vi "Configure System Time Stamp.vi"(7 "System Date Time":timestamp, 8 "error in (no error)":errorcluster, 9 "Time Stamp Format (0: Absolute)":i32(ring) items=["Absolute", "Delta"], 10 "Time Stamp Type (0: Relative-time)":i32(ring) items=["Relative-time", "Real-time"], 11 "VISA resource name":refnum<visa-resource-name>) -> (0 "error out":errorcluster, 3 "VISA resource name out":refnum<visa-resource-name>)   [LabVIEW 2020, in "Keithley 6517.lvlib"]
doc: "Configures time stamps.\n\nNote:\nFor relative-time time stamp, uses the values to set it only when disable reset relative time stamp.\n\nThis VI is <B>NOT</B> compatible with model <B>6514</B>."
uses:
  <instrlib>/Keithley 6517/Keithley 6517.lvlib
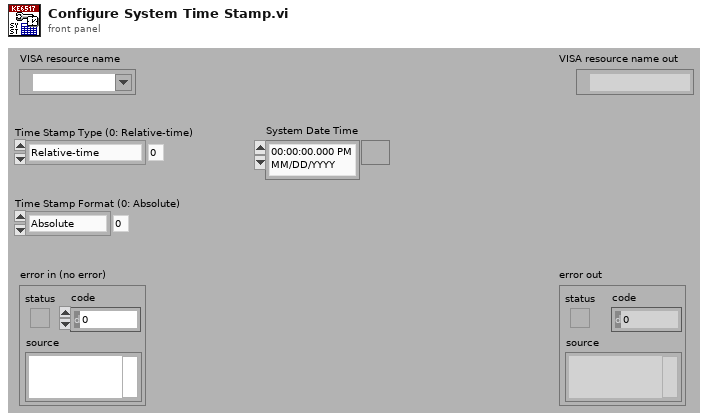
[diagram p1: front panel]
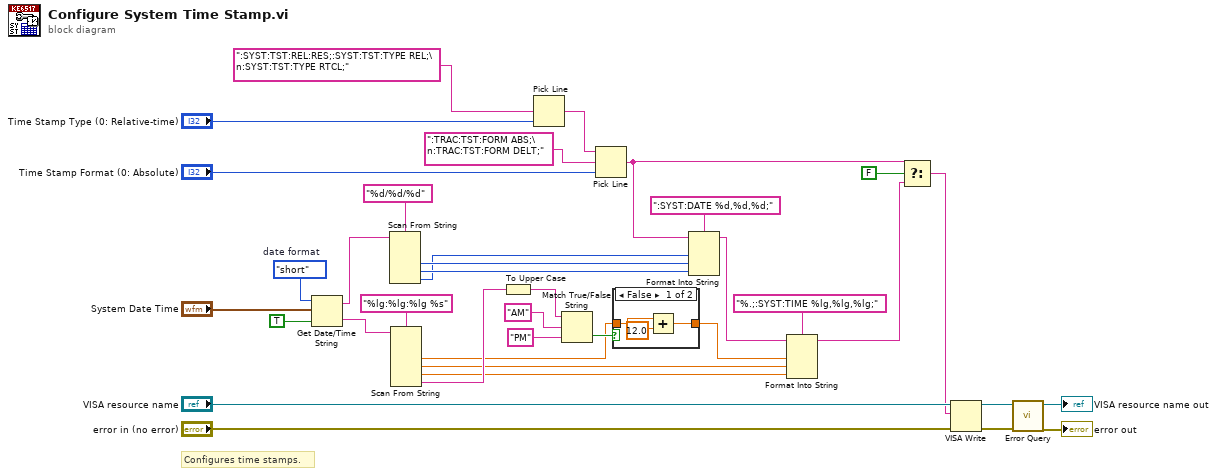
[diagram p0: block diagram]
diagram:
  w22 = enum16{"short", "long", "abbreviated"}."short"  # date format
  # "Configures time stamps."
  n1 = Get Date/Time String(date format (0)=w22, seconds (now)="System Date Time", want seconds? (F)=TRUE) -> (date string=w21:string, time string=w20:string)
  n2 = Scan From String(format string="%d/%d/%d", input string=w21) -> (output 1=w10:i32, output 2=w9:i32, output 3=w8:i32)  [unwired: 5 in, 3 out]
  n3 = Scan From String(format string="%lg:%lg:%lg %s", input string=w20) -> (output 1=w12:dbl, output 2=w6:dbl, output 3=w5:dbl, output 4=w17:string)  [unwired: 6 in, 3 out]
  n4 = To Upper Case(1:w17) -> (0:w16:string)
  n5 = Pick Line(multi-line string=":SYST:TST:REL:RES;:SYST:TST:TYPE REL;\n:SYST:TST:TYPE RTCL;", line index="Time Stamp Type (0: Relative-time)") -> (output string=w24:string)  [unwired: 1 in]
  n6 = Match True/False String(2:"PM" ("false string"), 3:"AM" ("true string"), 4:w16) -> (0:w13:bool)  [unwired: 1 out]
  n7 = Pick Line(string ("")=w24, multi-line string=":TRAC:TST:FORM ABS;\n:TRAC:TST:FORM DELT;", line index="Time Stamp Format (0: Absolute)") -> (output string=w2:string)
  n8 = case shown="False" w13 {
    tunnel: w12 -> [w39 w41]
    tunnel: [w40 w41] -> w7
    frame False {
      n9 = Add(x=w39, y=12.0) -> (x+y=w40:dbl)
    }
    frame True {
    }
  }
  n10 = Format Into String(format string=":SYST:DATE %d,%d,%d;", initial string=w2, w8, w10, w9) -> (resulting string=w36:string)  [unwired: 1 in, 1 out]
  n11 = Format Into String(format string="%.;:SYST:TIME %lg,%lg,%lg;", initial string=w36, w7, w6, w5) -> (resulting string=w3:string)  [unwired: 1 in, 1 out]
  n12 = Select(t=w2, s=FALSE, f=w3) -> (s? t:f=w4:string)
  n13 = VISA Write(VISA resource name="VISA resource name", write buffer=w4, error in (no error)="error in (no error)") -> (VISA resource name out=w32:refnum<visa-resource-name>, error out=w31:errorcluster)  [unwired: 1 out]
  n14 = call <instrlib>:"Error Query.vi"("error in (no error)"=w31, "VISA resource name"=w32) -> ("error out"=→"error out":errorcluster, "VISA resource name out"=→"VISA resource name out":refnum<visa-resource-name>)  [unwired: 6 in, 2 out]
